vi "RFmxSpecAn CHP (Analysis Only) with Recommended Settings.vi"() -> ()   [LabVIEW 2017]
doc: "This example illustrates how to use NI-RFmx in hardware agnostic mode to perform measurements on user provided IQ or Spectrum waveform. The example uses NI-RFSA driver API to acquire waveform from NI RF Signal Analyzer and perform an ACP measurement. The NI-RFSA acquisition settings are read from NI-RFmx session after Commit VI call. The NI-RFmx session is opened with Option String set as \"AnalysisOnly=1\"."
uses:
  <vilib>/Utility/error.llb/DialogType.ctl
  <vilib>/Analysis/1siggen.llb/Ramp Pattern by Delta.vi
  <instrlib>/niRFSA/niRFSA.llb/niRFSA Fetch IQ (1D Complex WDT NRec 1Chan).vi
  <vilib>/RFmx/SpecAn/mx/RFmxSpecAn.llb/RFmxSpecAn Analyze (IQ).vi
  <vilib>/RFmx/SpecAn/mx/RFmxSpecAn.llb/RFmxSpecAn CHP Fetch Measurement.vi
  <vilib>/Analysis/NI_AALBase.lvlib
  <vilib>/RFmx/SpecAn/mx/RFmxSpecAn.llb/RFmxSpecAn TXP Fetch Power Trace.vi
panel:
  in  "Resource Name LO Signal Generation":refnum<k15>="RFSG" caption="resource name"
  in  "Resource Name Test Signal Generation":refnum<k15>="RFSG" caption="resource name"
  in  "Stop Carrier Frequency (Hz)":dbl=6000000000.0 format="%#_6p"
  out "XY Graph":cluster{dbl[], dbl[]}(graph)
  in  "number of records":i64=50
  in  "Start Carrier Frequency (Hz)":dbl=4000000000.0 format="%#_6p"
  in  "Resource Name 2":refnum<k15>="RFSA" caption="Resource Name"
  in  "Reference Level (dBm)":dbl format="%.2f"
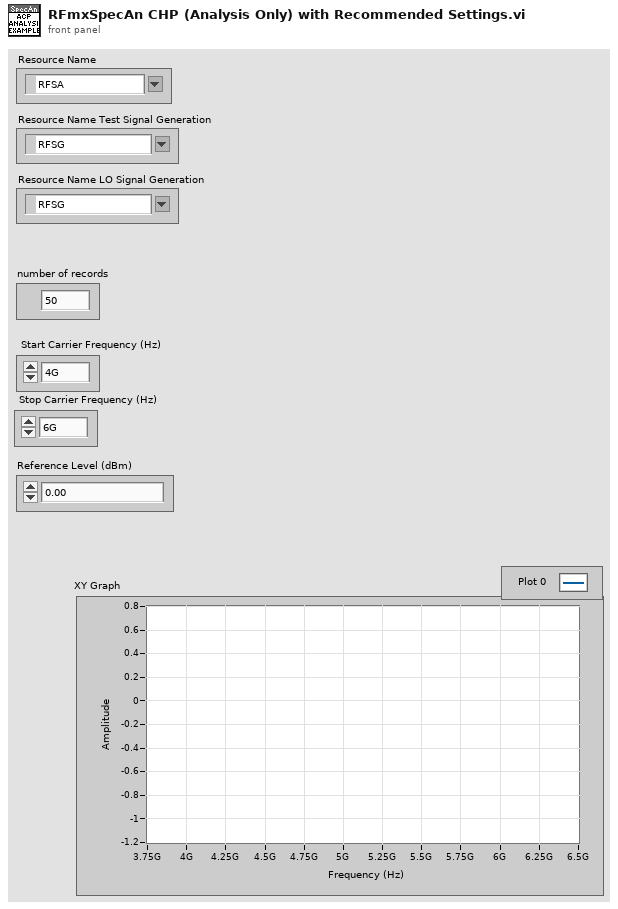
[diagram p1: front panel]
types:
  T1 = typedef "DialogType.ctl" = u16
  T2 = typedef "niRFmx Instrument Handle.ctl" = refnum<k21>
  T3 = enum16{"open", "open or create", "create or replace", "create", "open (read-only)"}
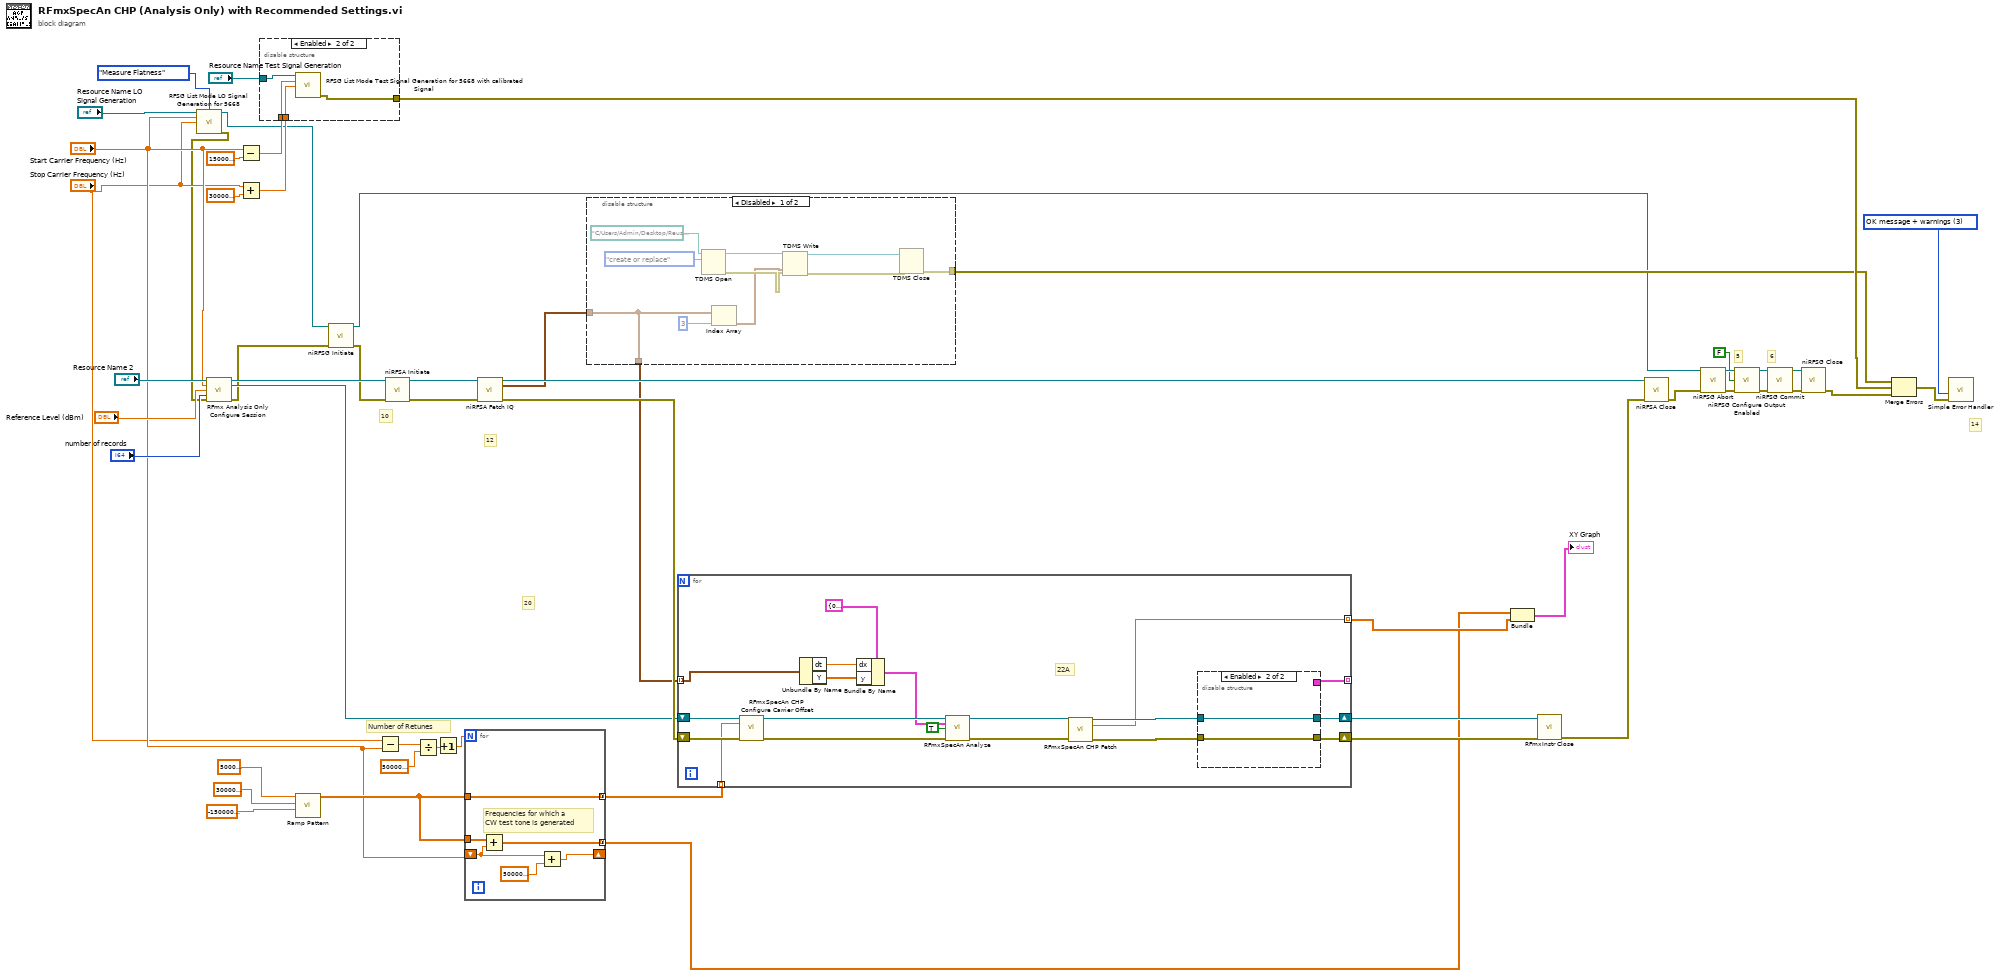
[diagram p0: block diagram]
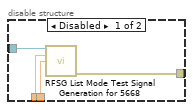
[diagram p2: hidden frame]
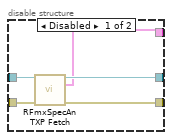
[diagram p4: hidden frame]
diagram:
  w52 = T1 3 items=["no dialog", "OK message", "continue or stop message", "OK message + warnings", "continue/stop + warnings"] ("type of dialog (OK msg:1)")
  # "6"
  # "5"
  # "Number of Retunes"
  # "12"
  # "10"
  # "14"
  # "20"
  n1 = call "RFSG List Mode LO Signal Generation for 5668.vi"("Resource Name"="Resource Name LO Signal Generation", "Mode"=enum16{"Normal", "Measure Flatness"}."Measure Flatness", "Start Frequency"="Start Carrier Frequency (Hz)", "End Frequency"="Stop Carrier Frequency (Hz)") -> ("instrument handle out"=w13:refnum<k15>, "error out"=w14:errorcluster)  [unwired: 10 in]
  n2 = call "RFmx Analysis Only Configure Session.vi"("IVI Refnum in"="Resource Name 2", "Carrier Frequency (Hz)"="Start Carrier Frequency (Hz)", "Reference Level (dBm)"="Reference Level (dBm)", "number of records"="number of records", "error in (no error)"=w14) -> ("RFSA Instrument Handle Out"=w49:refnum<k15>, "RFmx Instrument Handle Out"=w45:T2, "error out 2"=w12:errorcluster)  [unwired: 8 in]
  n3 = Subtract(x="Start Carrier Frequency (Hz)", y=150000000.0) -> (x-y=w34:dbl)
  n4 = Add(x="Stop Carrier Frequency (Hz)", y=300000000.0) -> (x+y=w33:dbl)
  n5 = disable-structure shown="Enabled" {
    disable-tunnel: w34 -> [w57 w60]
    disable-tunnel: w33 -> [w56 w59]
    disable-tunnel: "Resource Name Test Signal Generation" -> [w55 w61]
    disable-tunnel: [w54 w58] -> w31
    frame Disabled {
      n6 = call "RFSG List Mode Test Signal Generation for 5668.vi"("Resource Name"=w55, "Start Frequency"=w57, "End Frequency"=w56) -> ("error out"=w54:errorcluster)  [unwired: 11 in, 1 out]
    }
    frame Enabled {
      n7 = call "RFSG List Mode Test Signal Generation for 5668 with calibrated Signal.vi"("Resource Name"=w61, "Start Frequency"=w60, "End Frequency"=w59) -> ("error out"=w58:errorcluster)  [unwired: 11 in, 1 out]
    }
  }
  n8 = call-poly <vilib>:"Ramp Pattern.vi"("start"=-150000000.0, "end"=300000000.0, "delta"=50000000.0) -> ("Ramp Pattern"=w23:dbl[])  [unwired: 6 in, 2 out]
  n9 = call <instrlib>:"niRFSG Initiate.vi"("instrument handle"=w13, "error in"=w12) -> ("instrument handle out"=w1:refnum<k15>, "error out"=w11:errorcluster)  [unwired: 12 in]
  n10 = Subtract(x="Stop Carrier Frequency (Hz)", y="Start Carrier Frequency (Hz)") -> (x-y=w29:dbl)
  n11 = call <instrlib>:"niRFSA Initiate.vi"("instrument handle"=w49, "error in"=w11) -> ("instrument handle out"=w44:refnum<k15>, "error out"=w43:errorcluster)  [unwired: 12 in]
  n12 = Divide(x=w29, y=500000000.0) -> (x/y=w27:dbl)
  n13 = Increment(x=w27) -> (x+1=w26:dbl)
  n14 = for {
    N: w26 -> [_]
    tunnel: w23 -> [w67]
    tunnel: [w67] -> w25 mode=concatenating
    tunnel: w23 -> [w66]
    shift-right: [w63] -> _
    shift-left: "Start Carrier Frequency (Hz)" -> [w65]
    tunnel: [w62] -> w22 mode=concatenating
    # "Frequencies for which a \nCW test tone is generated"
    n15 = Add(x=w66, y=w65) -> (x+y=w62:dbl[])
    n16 = Add(x=w65, y=500000000.0) -> (x+y=w63:dbl)
  }
  n17 = call-poly <instrlib>:"niRFSA Fetch IQ.vi"("instrument handle"=w44, "error in"=w43) -> ("instrument handle out"=w51:refnum<k15>, "data"=w20:waveform(cdb)[], "error out"=w48:errorcluster)  [unwired: 11 in]
  n18 = disable-structure shown="Disabled" {
    disable-tunnel: [w71 _] -> w21
    disable-tunnel: w20 -> [w68 w78]
    disable-tunnel: [w68 w78] -> w19
    frame Disabled {
      n19 = TDMS Open(10:T3."create or replace" ("operation (0:open)"), 11:path "C:/Users/Admin/Desktop/Reuse/Scanning Speed PXIe 5668/Data8G.tdms.txt" ("file path")) -> (0:w75:errorcluster, 3:w74:refnum<k34>)  [unwired: 5 in]
      n20 = Index Array(array=w68, index=3) -> (element=w69:waveform(cdb))
      n21 = TDMS Write(0:w74, 9:w69, 11:w75) -> (4:w72:refnum<k34>, 15:w73:errorcluster)  [unwired: 3 in, 2 out]
      n22 = TDMS Close(8:w73, 11:w72) -> (0:w71:errorcluster)  [unwired: 1 out]
    }
    frame Enabled {
    }
  }
  n23 = for {
    shift-right: [w95] -> w46
    shift-left: w48 -> [w97]
    shift-right: [w96] -> w47
    shift-left: w45 -> [w84]
    tunnel: [w85] -> w39 mode=indexing
    tunnel: w19 -> [w83] mode=indexing
    tunnel: [w92] -> _ mode=indexing
    tunnel: w25 -> [w86] mode=indexing
    # "22A"
    n24 = call <vilib>:"RFmxSpecAn CHP Configure Carrier Offset.vi"("Instrument Handle In"=w84, "Carrier Frequency (Hz)"=w86, "error in (no error)"=w97) -> ("Instrument Handle Out"=w87:refnum<k21>, "error out"=w88:errorcluster)  [unwired: 11 in]
    n25 = Unbundle By Name(w83) -> ("dt"=w81:dbl, "Y"=w80:cdb[])
    n26 = Bundle By Name(cluster=cluster{"x0":dbl, "dx":dbl, "y":csg[]} {"x0"=0.0, "dx"=0.0, "y"=[]} ("IQ"), "dx"=w81, "y"=w80) -> (w79:cluster{"x0":dbl, "dx":dbl, "y":csg[]})
    n27 = call-poly <vilib>:"RFmxSpecAn Analyze.vi"("Instrument Handle In"=w87, "IQ"=w79, "Reset?"=TRUE, "error in (no error)"=w88) -> ("Instrument Handle Out"=w91:refnum<k21>, "error out"=w90:errorcluster)  [unwired: 8 in, 2 out]
    n28 = call-poly <vilib>:"RFmxSpecAn CHP Fetch.vi"("Instrument Handle In"=w91, "error in (no error)"=w90) -> ("Instrument Handle Out"=w89:refnum<k21>, "Absolute Power (dBm)"=w85:dbl, "error out"=w93:errorcluster)  [unwired: 8 in, 3 out]
    n29 = disable-structure shown="Enabled" {
      disable-tunnel: [w102 w104] -> w96
      disable-tunnel: [w101 w103] -> w95
      disable-tunnel: w93 -> [w100 w103]
      disable-tunnel: [w99 _] -> w92
      disable-tunnel: w89 -> [w98 w104]
      frame Disabled {
        n30 = call-poly <vilib>:"RFmxSpecAn TXP Fetch.vi"("Instrument Handle In"=w98, "error in (no error)"=w100) -> ("Instrument Handle Out"=w102:refnum<k21>, "Power (dBm)"=w99:cluster{"x0":dbl, "dx":dbl, "y":sgl[]}, "error out"=w101:errorcluster)  [unwired: 11 in]
      }
      frame Enabled {
      }
    }
  }
  n31 = Bundle(w22, w39) -> (→"XY Graph":cluster{dbl[], dbl[]})  [unwired: 1 in]
  n32 = call <vilib>:"RFmxInstr Close.vi"("Instrument Handle In"=w47, "error in (no error)"=w46) -> ("error out"=w53:errorcluster)  [unwired: 13 in]
  n33 = call <instrlib>:"niRFSA Close.vi"("instrument handle"=w51, "error in"=w53) -> ("error out"=w4:errorcluster)  [unwired: 13 in]
  n34 = call <instrlib>:"niRFSG Abort.vi"("instrument handle"=w1, "error in"=w4) -> ("instrument handle out"=w9:refnum<k15>, "error out"=w10:errorcluster)  [unwired: 12 out]
  n35 = call <instrlib>:"niRFSG Configure Output Enabled.vi"("instrument handle"=w9, "output enabled"=FALSE ("output enable"), "error in"=w10) -> ("instrument handle out"=w5:refnum<k15>, "error out"=w6:errorcluster)  [unwired: 11 out]
  n36 = call <instrlib>:"niRFSG Commit.vi"("instrument handle"=w5, "error in"=w6) -> ("instrument handle out"=w8:refnum<k15>, "error out"=w7:errorcluster)  [unwired: 12 out]
  n37 = call <instrlib>:"niRFSG Close.vi"("instrument handle"=w8, "error in"=w7) -> ("error out"=w3:errorcluster)  [unwired: 13 out]
  n38 = Merge Errors(w21, w31, w3) -> (w30:errorcluster)
  n39 = call <vilib>:"Simple Error Handler.vi"("type of dialog (OK msg:1)"=w52, "error in (no error)"=w30) -> ()  [unwired: 3 in, 5 out]
